vi "WPI_MXP DIO Channel to MXP Pin.vi"(7 "DIOChannel":T1) -> (8 "Shared MXP Pin":T2)   [LabVIEW 2017]
uses:
  <vilib>/Rock Robotics/WPI/MXP/WPI_MXP Shared MXP Pin.ctl
  <vilib>/Rock Robotics/SystemInterfaces/DIO/FPGA_DIOChannel.ctl
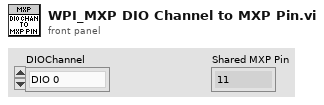
[diagram p1: front panel]
types:
  T1 = typedef "FPGA_DIOChannel.ctl" = enum8{"DIO 0", "DIO 1", "DIO 2", "DIO 3", "DIO 4", "DIO 5", "DIO 6", "DIO 7", "DIO 8", "DIO 9", "DIO MXP 0", "DIO MXP 1", "DIO MXP 2", "DIO MXP 3", "DIO MXP 4", "DIO MXP 5", "DIO MXP 6", "DIO MXP 7", "DIO MXP 8", "DIO MXP 9", "DIO MXP 10", "DIO MXP 11", "DIO MXP 12", "DIO MXP 13", "DIO MXP 14", "DIO MXP 15", "SPI Port CS1", "SPI Port CS2", "SPI Port CS3", "SPI Port MISO", "SPI Port MOSI", "Invalid"}
  T2 = typedef "WPI_MXP Shared MXP Pin.ctl" = enum16{"11", "13", "15", "17", "19", "21", "23", "25", "27", "29", "31", "18", "22", "26", "32", "34", "Invalid"}
  T3 = enum16{"11", "13", "15", "17", "19", "21", "23", "25", "27", "29", "31", "18", "22", "26", "32", "34", "Invalid"}
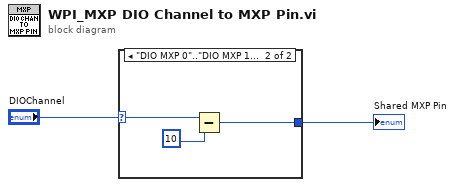
[diagram p0: block diagram]
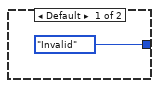
[diagram p2: hidden frame]
diagram:
  n1 = case shown="\"DIO MXP 0\"..\"DIO MXP 15\"" "DIOChannel" {
    selector: "DIOChannel" -> [_ w6]
    tunnel: [T3."Invalid" ("Shared MXP Pin") w4] -> w1
    frame Default {
    }
    frame "DIO MXP 0".."DIO MXP 15" {
      n2 = Subtract(x=w6, y=u8 10) -> (x-y=w4:u8)
    }
  }
  "Shared MXP Pin" <- w1
